vi "COM Curent Read.vi"(8 "error in (no error)":errorcluster, 10 "VI reference (current VI)":refnum<vi>, 11 "VISA resource name 2":refnum<visa-resource-name>) -> (0 "error out":errorcluster, 2 ".not. x?":bool, 3 "VISA Current":refnum<visa-resource-name>)   [LabVIEW 2017]
uses:
  <vilib>/Instr/_visa.llb/VISA Configure Serial Port (Instr).vi
panel:
  in  "Blank Button":bool
  in  "VISA resource name":refnum<visa-resource-name>
  # "Please choose the Curent COM Port"
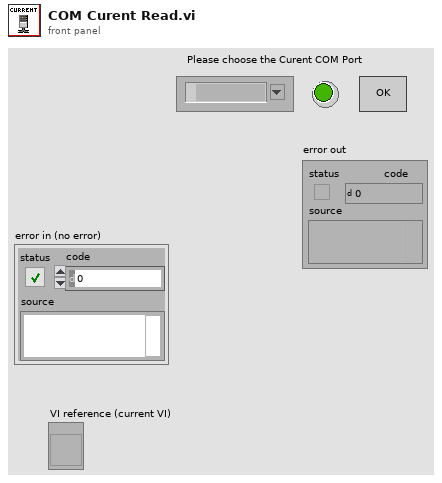
[diagram p1: front panel]
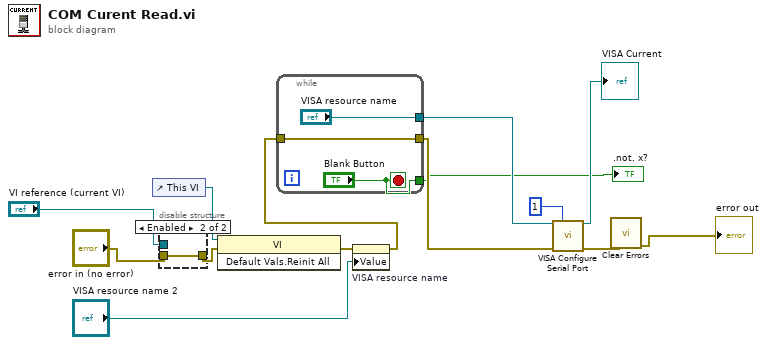
[diagram p0: block diagram]
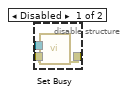
[diagram p2: hidden frame]
diagram:
  n1 = control-ref of="This VI"() -> (w14:refnum<vi>)
  n2 = disable-structure shown="Enabled" {
    disable-tunnel: "VI reference (current VI)" -> [w17 _]
    disable-tunnel: "error in (no error)" -> [w16 w18]
    disable-tunnel: [w15 w18] -> w6
    frame Disabled {
      n3 = call <vilib>:"Set Busy.vi"("error in (no error)"=w16, "VI reference (current VI)"=w17) -> ("error out"=w15:errorcluster)  [unwired: 8 in, 1 out]
    }
    frame Enabled {
    }
  }
  n4 = invoke class="VI" method="Default Vals.Reinit All"(reference=w14, error in=w6) -> (error out=w13:errorcluster)  [unwired: 1 in, 2 out]
  n5 = property on="VISA resource name" class="VISAName"(error in=w13, "Value"="VISA resource name 2") -> (error out=w5:errorcluster)  [unwired: 1 in, 1 out]
  n6 = while {
    tunnel: ["VISA resource name"] -> w11
    tunnel: w5 -> [w20]
    tunnel: [w20] -> w4
    tunnel: ["Blank Button"] -> w2
    stop <- "Blank Button" stop-if-true
  }
  ".not. x?" <- w2
  n7 = call-poly "VISA Configure Serial Port"("VISA resource name"=w11, "timeout (10sec)"=u32 1, "error in (no error)"=w4) -> ("VISA resource name out"=→"VISA Current":refnum<visa-resource-name>, "error out"=w1:errorcluster)  [unwired: 11 in]
  n8 = call <vilib>:"Clear Errors.vi"("error in (no error)"=w1) -> ("error out"=→"error out":errorcluster)  [unwired: 5 in, 1 out]
